vi "TriggerDeadzone.vi"(11 "upper limit in":dbl) -> (3 "upper limit out":dbl)   [LabVIEW 2014]
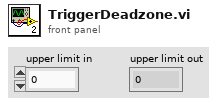
[diagram p1: front panel]
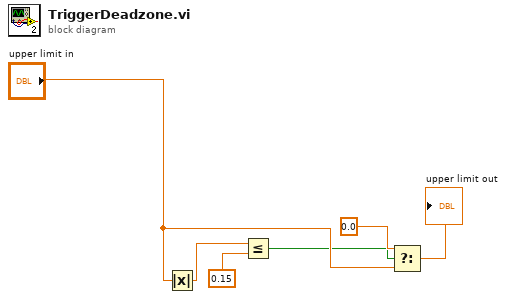
[diagram p0: block diagram]
diagram:
  n1 = Absolute Value(x="upper limit in") -> (abs(x)=w1:dbl)
  n2 = Less Or Equal?(x=w1, y=0.15) -> (x <= y?=w3:bool)
  n3 = Select(t=0.0, s=w3, f="upper limit in") -> (s? t:f=→"upper limit out":dbl)
